vi "Get Status.vi"(11 "error in":errorcluster) -> (3 "Gripper SP":cluster{"Left":dbl, "Right":dbl}, 4 "Elevator Sensor":dbl, 6 "Gripper Sensor":cluster{"Left":dbl, "Right":dbl}, 8 "Elevator Moving?":bool, 10 "Gripper Moving?":bool, 14 "Elevator SP":dbl, 15 "error out":errorcluster)   [LabVIEW 2014, in "Elevator System.lvlib"]
uses:
  Elevator System.lvlib
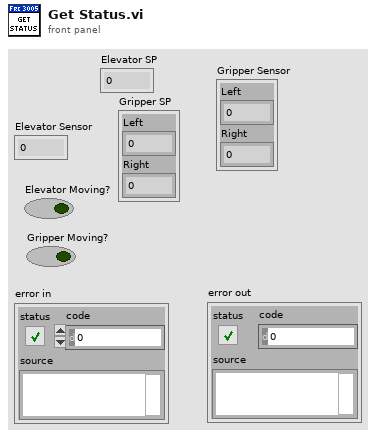
[diagram p1: front panel]
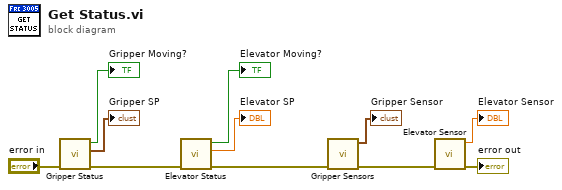
[diagram p0: block diagram]
diagram:
  n1 = call "Gripper Status.vi"("error in"="error in") -> ("error out"=w6:errorcluster, "Gripper SP"=→"Gripper SP":cluster{"Left":dbl, "Right":dbl}, "Moving?"=→"Gripper Moving?":bool)  [unwired: 8 in]
  n2 = call "Elevator Status.vi"("error in"=w6) -> ("error out"=w5:errorcluster, "Elevator SP"=→"Elevator SP":dbl, "Moving?"=→"Elevator Moving?":bool)  [unwired: 8 in]
  n3 = call "Gripper Sensors.vi"("error in"=w5) -> ("error out"=w4:errorcluster, "Gripper Values"=→"Gripper Sensor":cluster{"Left":dbl, "Right":dbl})  [unwired: 9 in]
  n4 = call "Elevator Sensor.vi"("error in"=w4) -> ("error out"=→"error out":errorcluster, "Value"=→"Elevator Sensor":dbl)  [unwired: 9 in]
